vi "Latency Round Trip Example.vi"() -> ()   [LabVIEW 2020]
uses:
  Controls/Backends.ctl
  Controls/Audio Device Info.ctl
  Controls/Audio Device Type.ctl
  Controls/Audio Device Native Data Format.ctl
  Controls/Audio Device Format.ctl
  Controls/Latency Test Config.ctl
  Controls/Latency Test Device Config.ctl
  Controls/Audio Device Config.ctl
  Controls/Audio Device Advanced Config.ctl
  Controls/Latency Test Message.ctl
  Controls/Latency Test Loopback State.ctl
  G-Audio.lvlib
panel:
  out "Audio State":string
  out "Actual Config":T1={"Backend"=enum."Default", "Read / Write Buffer"=1024, "Capture Device"={"Name"=0, "ID"=[], "Buffer Size"=4096, "Config"={"Sample Rate (Hz)"=44100, "Channels"=2, "Format"=enum."I16"}, "Advanced Config"={"Exclusive Mode"=FALSE, "Period Size"=0, "Num Periods"=0, "Optimize Latency"=FALSE}}, "Playback Device"={"Name"=0, "ID"=[], "Buffer Size"=4096, "Config"={"Sample Rate (Hz)"=44100, "Channels"=2, "Format"=enum."I16"}, "Advanced Config"={"Exclusive Mode"=FALSE, "Period Size"=0, "Num Periods"=0, "Optimize Latency"=FALSE}}} {"Playback Device"."Name" items=["Primary Sound Capture Driver", "Microphone (High Definition Audio Device)"]; "Capture Device"."Name" items=["Primary Sound Driver", "Speakers (High Definition Audio Device)"]}
  out "error out":errorcluster
  in  "Config":T1={"Backend"=enum."WASAPI", "Read / Write Buffer"=1024, "Capture Device"={"Name"=0, "ID"=[123, 0, 48, 0, 46, 0, 48, 0, 46, 0, 49, 0, 46, 0, 48, 0, 48, 0, 48, 0, 48, 0, 48, 0, 48, 0, 48, 0, 48, 0, 125, 0, 46, 0, 123, 0, 101, 0, 52, 0, 51, 0, 51, 0, 54, 0, 56, 0, 101, 0, 52, 0, 45, 0, 54, 0, 51, 0, 97, 0, 100, 0, 45, 0, 52, 0, 57, 0, 53, 0, 100, 0, 45, 0, 57, 0, 100, 0, 50, 0, 50, 0, 45, 0, 52, 0, 52, 0, 55, 0, 52, 0, 98, 0, 100, 0, 101, 0, 50, 0, 101, 0, 50, 0, 57, 0, 55, 0, 125, 0, 0, 0, 0, 0, 0, 0, 0, 0, 0, 0, 0, 0, 0, 0, 0, 0, 0, 0, 0, 0, 0, 0, 0, 0, 0, 0, 0, 0, 0, 0, 0, 0, 0, 0, 0, 0, 0, 0, 0, 0, 0, 0, 0, 0, 0, 0, 0, 0, 0, 0, 0, 0, 0, 0, 0, 0, 0, 0, 0, 0, 0, 0, 0, 0, 0, 0, 0, 0, 0, 0, 0, 0, 0, 0, 0, 0, 0, 0, 0, 0, 0, 0, 0, 0, 0, 0, 0, 0, 0, 0, 0, 0, 0, 0, 0, 0, 0, 0, 0, 0, 0, 0, 0, 0, 0, 0, 0, 0, 0, 0, 0, 0, 0, 0, 0, 0, 0, 0, 0, 0, 0, 0, 0, 0, 0, 0, 0, 0, 0, 0, 0, 0, 0, 0, 0, 0, 0, 0, 0, 0, 0, 0, 0, 0, 0, 0], "Buffer Size"=4096, "Config"={"Sample Rate (Hz)"=44100, "Channels"=2, "Format"=enum."I16"}, "Advanced Config"={"Exclusive Mode"=FALSE, "Period Size"=0, "Num Periods"=0, "Optimize Latency"=FALSE}}, "Playback Device"={"Name"=0, "ID"=[123, 0, 48, 0, 46, 0, 48, 0, 46, 0, 48, 0, 46, 0, 48, 0, 48, 0, 48, 0, 48, 0, 48, 0, 48, 0, 48, 0, 48, 0, 125, 0, 46, 0, 123, 0, 53, 0, 98, 0, 48, 0, 51, 0, 99, 0, 100, 0, 54, 0, 49, 0, 45, 0, 97, 0, 50, 0, 53, 0, 53, 0, 45, 0, 52, 0, 97, 0, 101, 0, 53, 0, 45, 0, 97, 0, 51, 0, 51, 0, 101, 0, 45, 0, 52, 0, 98, 0, 100, 0, 102, 0, 99, 0, 53, 0, 101, 0, 101, 0, 57, 0, 51, 0, 102, 0, 55, 0, 125, 0, 0, 0, 0, 0, 0, 0, 0, 0, 0, 0, 0, 0, 0, 0, 0, 0, 0, 0, 0, 0, 0, 0, 0, 0, 0, 0, 0, 0, 0, 0, 0, 0, 0, 0, 0, 0, 0, 0, 0, 0, 0, 0, 0, 0, 0, 0, 0, 0, 0, 0, 0, 0, 0, 0, 0, 0, 0, 0, 0, 0, 0, 0, 0, 0, 0, 0, 0, 0, 0, 0, 0, 0, 0, 0, 0, 0, 0, 0, 0, 0, 0, 0, 0, 0, 0, 0, 0, 0, 0, 0, 0, 0, 0, 0, 0, 0, 0, 0, 0, 0, 0, 0, 0, 0, 0, 0, 0, 0, 0, 0, 0, 0, 0, 0, 0, 0, 0, 0, 0, 0, 0, 0, 0, 0, 0, 0, 0, 0, 0, 0, 0, 0, 0, 0, 0, 0, 0, 0, 0, 0, 0, 0, 0, 0, 0, 0], "Buffer Size"=4096, "Config"={"Sample Rate (Hz)"=44100, "Channels"=2, "Format"=enum."I16"}, "Advanced Config"={"Exclusive Mode"=FALSE, "Period Size"=0, "Num Periods"=0, "Optimize Latency"=FALSE}}} {"Playback Device"."Name" items=["Speakers (High Definition Audio Device)"]; "Capture Device"."Name" items=["Microphone (High Definition Audio Device)"]}
  in  "Run":bool
  out "Capture Devices":T7[](array[typedef])
  out "Playback Devices":T7[](array[typedef])
  in  "Query Devices":bool
  in  "Backend":T2
  # "Instructions:\n1. Run the VI.\n2. On the left select a Backend, then click Query Devices to populate the Capture and Playback device lists.\n3. In the configuration section on the right, select the name of the Capture and Playback device to be used.\n4. Adjust the configuration of each device and the Read / Write Buffer size, then press Run Capture + Playback.\n5. Audio from the capture device will be read and copied to the playback device. The amount of audio data copied per iteration is determined by Read / Write Buffer.\n\nLatency reduction tips:\n1. Use identical sample rates, channels, formats, and period sizes for both capture and playback to avoid type conversions and waiting for buffers to fill.\n2. Use exclusive mode to avoid sample rate conversion and other processing performed by the backend / OS (WASAPI only).\n3. Use the same Read / Write Buffer size as the period size. Note this should be the actual period size after configuring the device. This size may not be what was requested, especially when not running in exclusive mode.\n4. The Optimize latency setting won't reduce latency by itself, but will run the backend capture / playback threads at a higher priority so smaller buffer sizes can be used while avoiding dropouts. (WASAPI only)"
  # "G"
  # "-Audio"
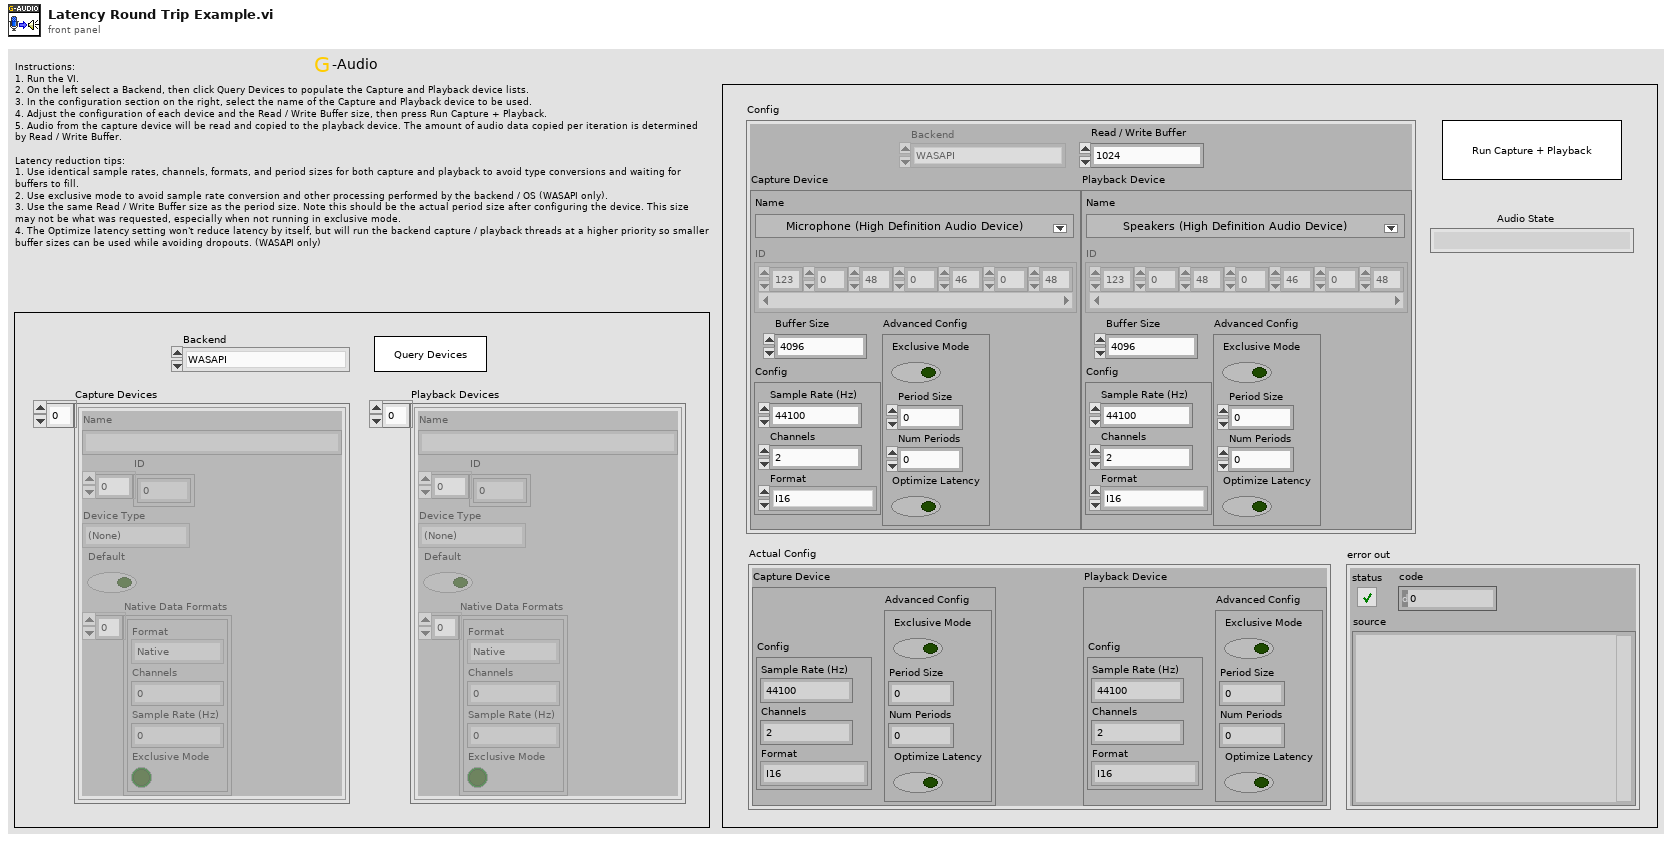
[diagram p1: front panel]
types:
  T1 = typedef "Latency Test Config.ctl" = cluster{"Backend":T2, "Read / Write Buffer":i32, "Capture Device":T3, "Playback Device":T3}
  T2 = typedef "G-Audio.lvlib/Backends.ctl" = enum16{"WASAPI", "DirectSound", "WinMM", "Core Audio", "sndio", "audio(4)", "OSS", "PulseAudio", "ALSA", "JACK", "AAudio", "OpenSL|ES", "Web Audio", "Custom", "Null", "Default"}
  T3 = typedef "Latency Test Device Config.ctl" = cluster{"Name":u16, "ID":u8[], "Buffer Size":u32, "Config":T4, "Advanced Config":T6}
  T4 = typedef "G-Audio.lvlib/Audio Device Config.ctl" = cluster{"Sample Rate (Hz)":u32, "Channels":u32, "Format":T5}
  T5 = typedef "G-Audio.lvlib/Audio Device Format.ctl" = enum16{"Native", "U8", "I16", "I32", "SGL"}
  T6 = typedef "G-Audio.lvlib/Audio Device Advanced Config.ctl" = cluster{"Exclusive Mode":bool, "Period Size":u32, "Num Periods":u32, "Optimize Latency":bool}
  T7 = typedef "G-Audio.lvlib/Audio Device Info.ctl" = cluster{"Name":string, "ID":u8[], "Device Type":T8, "Default":bool, "Native Data Formats":T9[]}
  T8 = typedef "G-Audio.lvlib/Audio Device Type.ctl" = enum16{"(None)", "Playback", "Capture", "Duplex", "Loopback"}
  T9 = typedef "G-Audio.lvlib/Audio Device Native Data Format.ctl" = cluster{"Format":T5, "Channels":u32, "Sample Rate (Hz)":u32, "Exclusive Mode":bool}
  T10 = typedef "Latency Test Message.ctl" = cluster{"Info":string, "Data":variant}
  T11 = enum32{"invalid app kind", "Development System", "Run Time System", "Student Edition", "Embedded LabVIEW", "Evaluation", "Custom"}
  T12 = typedef "Latency Test Loopback State.ctl" = enum16{"Idle", "Init", "Loopback", "Stop", "Shutdown", "Error"}
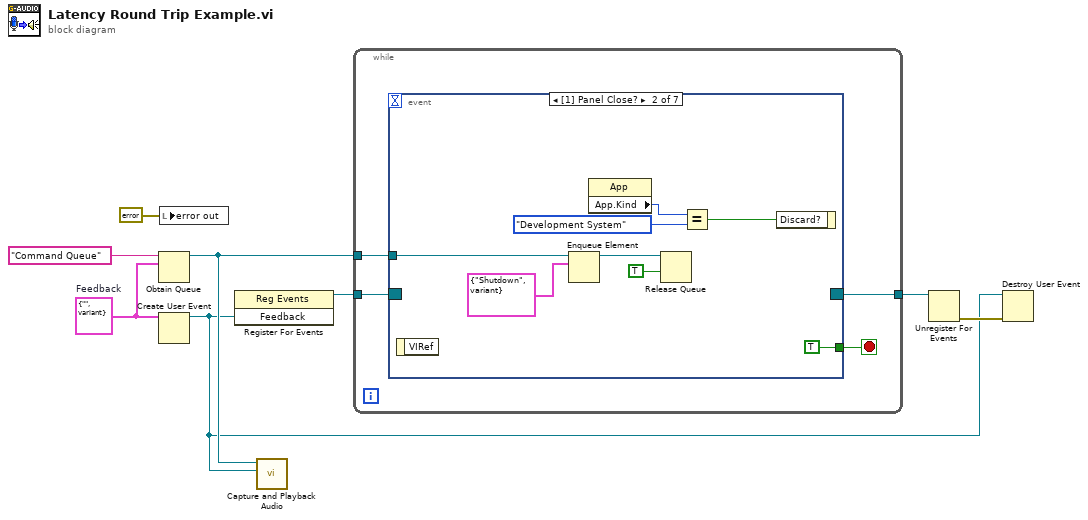
[diagram p0: block diagram]
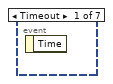
[diagram p2: hidden frame]
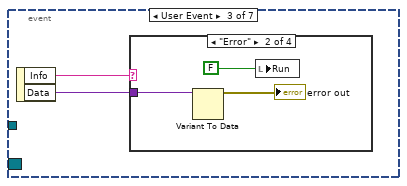
[diagram p3: hidden frame]
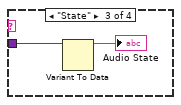
[diagram p5: hidden frame]
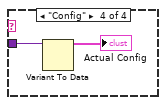
[diagram p6: hidden frame]
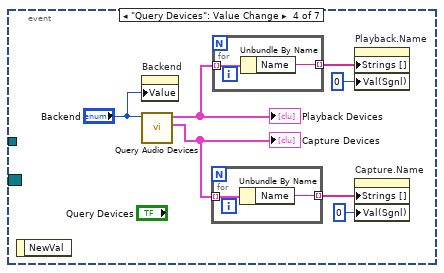
[diagram p7: hidden frame]
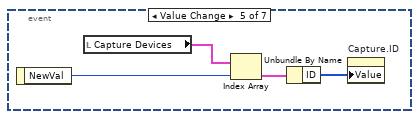
[diagram p8: hidden frame]
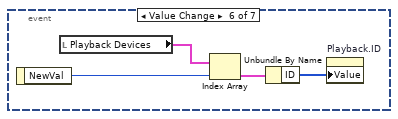
[diagram p9: hidden frame]
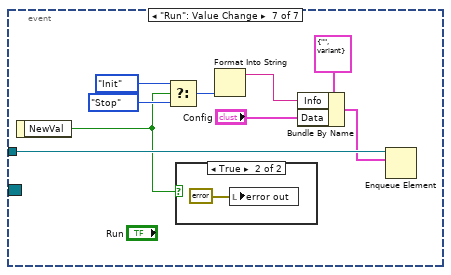
[diagram p10: hidden frame]
diagram:
  w7 = T10 {"Info"="", "Data"=variant}  # Feedback
  n1 = Obtain Queue(name (unnamed)="Command Queue", element data type=w7) -> (queue out=w5:refnum<queue>)  [unwired: 3 in, 2 out]
  n2 = Create User Event(user event datatype=w7) -> (user event=w2:refnum<user-event>)  [unwired: 1 in, 1 out]
  n3 = local write "error out"(errorcluster {"status"=FALSE, "code"=0, "source"=""} ("error out")) -> ()
  n4 = register-events(w2) -> (reference out=w8:refnum<event-registration>)  [unwired: 2 in, 1 out]
  n5 = call "Capture and Playback Audio.vi"("Feedback Event"=w2, "Command Queue"=w5) -> ()  [unwired: 10 in]
  n6 = while {
    tunnel: w8 -> [w11]
    tunnel: w5 -> [w10]
    tunnel: [w9] -> w3
    stop <- w12 stop-if-true
    n7 = event shown="[1] Panel Close?" {
      selector: w11 -> [_ _ _ _ _ _ _]
      dyn-events: [_ _ _ _ _ _ _] -> w9
      timeout: _ -> [_ _ _ _ _ _ _]
      tunnel: [_ TRUE _ _ _ _ _] -> w12
      tunnel: w10 -> [_ w14 _ _ _ _ w57]
      event Timeout {
        n8 = event-data() -> ()  [unwired: 1 in, 1 out]
      }
      event Panel Close? {
        n9 = event-data() -> ()  [unwired: 1 in, 1 out]
        n10 = Enqueue Element(queue=w14, element=T10 {"Info"="Shutdown", "Data"=variant}) -> (queue out=w15:refnum<queue>)  [unwired: 2 in, 2 out]
        n11 = property class="App"() -> ("App.Kind"=w20:T11)  [unwired: 2 in, 2 out]
        n12 = Release Queue(queue=w15, force destroy? (F)=TRUE) -> ()  [unwired: 1 in, 3 out]
        n13 = Equal?(x=w20, y=T11."Development System") -> (x = y?=w18:bool)
        n14 = event-data("Discard?"=w18) -> ()  [unwired: 1 in, 1 out]
      }
      event User Event {
        n15 = event-data() -> ("Info"=w22:string, "Data"=w21:variant)  [unwired: 1 in]
        n16 = case shown="\"Error\"" w22 {
          tunnel: w21 -> [_ w25 w27 w29]
          frame Default {
          }
          frame "Error" {
            n17 = Variant To Data(Variant=w25) -> (data=→"error out":errorcluster)  [unwired: 2 in, 1 out]
            n18 = local write "Run"(FALSE ("Run Loopback")) -> ()
          }
          frame "State" {
            n19 = Variant To Data(Variant=w27) -> (data=→"Audio State":string)  [unwired: 2 in, 1 out]
          }
          frame "Config" {
            n20 = Variant To Data(Variant=w29) -> (data=→"Actual Config":T1)  [unwired: 2 in, 1 out]
          }
        }
      }
      event "Query Devices": Value Change {
        n21 = event-data() -> ()  [unwired: 1 in, 1 out]
        n22 = property on="Backend" class="Enum (strict)"("Value"="Backend") -> ()  [unwired: 2 in, 2 out]
        n23 = call "Query Audio Devices.vi"("Backend (Default)"="Backend") -> ("Capture Devices"=w35:T7[], "Playback Devices"=w36:T7[])  [unwired: 6 in, 3 out]
        "Playback Devices" <- w36
        "Capture Devices" <- w35
        n24 = for {
          tunnel: w35 -> [w38] mode=indexing
          tunnel: [w37] -> w31 mode=indexing
          n25 = Unbundle By Name(w38) -> ("Name"=w37:string)
        }
        n26 = for {
          tunnel: w36 -> [w40] mode=indexing
          tunnel: [w39] -> w30 mode=indexing
          n27 = Unbundle By Name(w40) -> ("Name"=w39:string)
        }
        n28 = property on="Playback.Name" class="Ring (strict)"("Strings []"=w30, "Val(Sgnl)"=u16 0 ("Value (Signaling)")) -> ()  [unwired: 2 in, 2 out]
        n29 = property on="Capture.Name" class="Ring (strict)"("Strings []"=w31, "Val(Sgnl)"=u16 0 ("Value (Signaling)")) -> ()  [unwired: 2 in, 2 out]
      }
      event Value Change {
        n30 = event-data() -> ("NewVal"=w44:u16)  [unwired: 1 in]
        n31 = local read "Capture Devices"() -> (w43:T7[])
        n32 = Index Array(array=w43, index=w44) -> (element=w42:T7)
        n33 = Unbundle By Name(w42) -> ("ID"=w41:u8[])
        n34 = property on="Capture.ID" class="Arr (strict)"("Value"=w41) -> ()  [unwired: 2 in, 2 out]
      }
      event Value Change {
        n35 = event-data() -> ("NewVal"=w48:u16)  [unwired: 1 in]
        n36 = local read "Playback Devices"() -> (w47:T7[])
        n37 = Index Array(array=w47, index=w48) -> (element=w46:T7)
        n38 = Unbundle By Name(w46) -> ("ID"=w45:u8[])
        n39 = property on="Playback.ID" class="Arr (strict)"("Value"=w45) -> ()  [unwired: 2 in, 2 out]
      }
      event "Run": Value Change {
        n40 = event-data() -> ("NewVal"=w49:bool)  [unwired: 1 in]
        n41 = Select(t=Latency_Test_Loopback_State."Init" ("Loopback State"), s=w49, f=Latency_Test_Loopback_State."Stop") -> (s? t:f=w52:T12)
        n42 = case shown="True" w49 {
          frame False {
          }
          frame True {
            n43 = local write "error out"(errorcluster {"status"=FALSE, "code"=0, "source"=""} ("error out")) -> ()
          }
        }
        n44 = Format Into String(w52) -> (resulting string=w54:string)  [unwired: 3 in, 1 out]
        n45 = Bundle By Name(cluster=T10 {"Info"="", "Data"=variant} ("element"), "Info"=w54, "Data"="Config") -> (w55:T10)
        n46 = Enqueue Element(queue=w57, element=w55) -> ()  [unwired: 2 in, 3 out]
      }
    }
  }
  n47 = Unregister For Events(event registration refnum=w3) -> (error out=w4:errorcluster)  [unwired: 1 in]
  n48 = Destroy User Event(user event=w2, error in=w4) -> ()  [unwired: 1 out]
